vi "Init.vi"(8 "error in (no error)":errorcluster, 11 "Input Kind (All)":string) -> (0 "error out":errorcluster, 3 "GetInputList out":refnum<class "GetInputList.lvclass">)   [LabVIEW 2020, in "obs-websocket.lvlib" / "GetInputList.lvclass"]
uses:
  GetInputList.lvclass
  GetInputList.lvclass/GetInputList.ctl
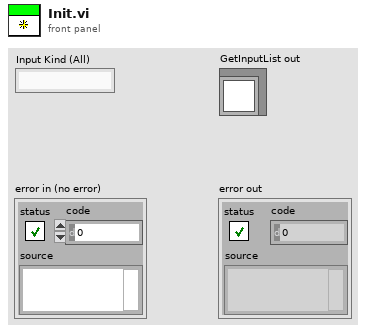
[diagram p1: front panel]
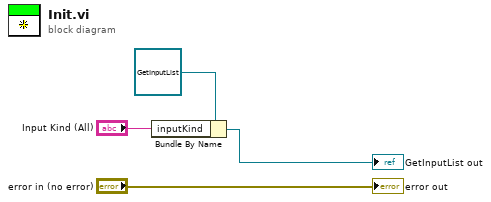
[diagram p0: block diagram]
diagram:
  n1 = Bundle By Name(cluster=refnum<class "GetInputList.lvclass"> refnum ("GetInputList in"), "inputKind"="Input Kind (All)") -> (→"GetInputList out":refnum<class "GetInputList.lvclass">)
  "error out" <- "error in (no error)"
